vi "Autonomous Independent.vi"() -> ()   [LabVIEW 2017]
doc: "This VI is called when autonomous begins, and will automatically be terminated when autonomous ends. You can carry out timed or sensor driven robot movement independently without needing to return to the caller."
uses:
  <vilib>/Rock Robotics/WPI/Utilities/WPI_GetSetVariantRefNum.vi
  <vilib>/Rock Robotics/Network Tables/NT Read String.vi
  <vilib>/Rock Robotics/WPI/RobotDrive/WPI_RobotDriveArcadeDrive_Standard(NoSaturation).vi
  <vilib>/Rock Robotics/Network Tables/NT Write Numeric Array.vi
  Robot Global Data.vi
panel:
  out "Current Movement, for debugging":T1 {"Y Joystick Value" scale=1.0..-1.0; "X Joystick Value" scale=-1.0..1.0}
  in  "Array of robot movements":T2(array[cluster])=[{"X Joystick Value"=0.39393939393939403, "Y Joystick Value"=0.0, "Delay (sec)"=1.0, "Movement Name"="turn"}, {"X Joystick Value"=-0.3737373737373737, "Y Joystick Value"=0.0, "Delay (sec)"=1.0, "Movement Name"="turn back"}] {"Y Joystick Value" scale=1.0..-1.0; "X Joystick Value" scale=-1.0..1.0}
  # "Be sure to right-click and choose Data Operations>>Make Current Value default if you want to save the array values with the VI"
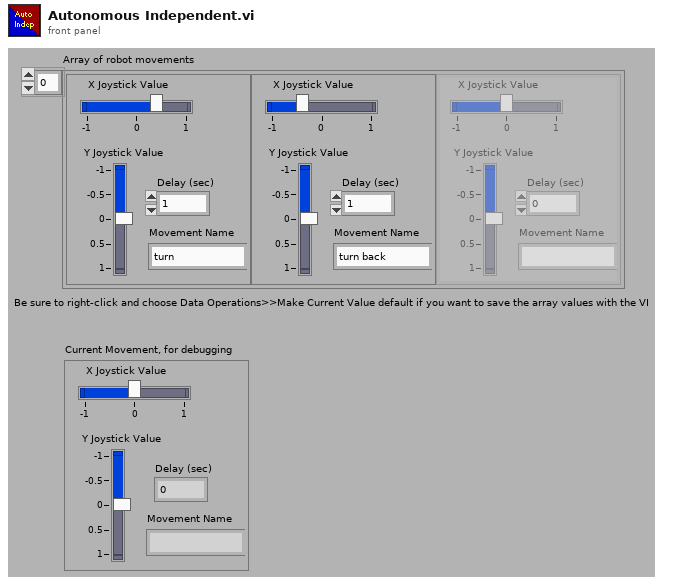
[diagram p1: front panel]
types:
  T1 = cluster{"X Joystick Value":dbl, "Y Joystick Value":dbl, "Delay (sec)":dbl, "Movement Name":string}
  T2 = cluster{"X Joystick Value":dbl, "Y Joystick Value":dbl, "Delay (sec)":dbl, "Movement Name":string}[]
  T3 = typedef "WPI_JoystickDevRef.ctl" = cluster{"Device":T4}
  T4 = typedef "WPI_JoystickDeviceEnum.ctl" = enum16{"USB 0", "USB 1", "USB 2", "USB 3", "USB 4", "USB 5"}
  T5 = typedef "WPI_EncoderDevRef.ctl" = cluster{"DevStatus":errorcluster, "EncoderIndex":T6, "CounterIndex":T7, "DistancePerCount":dbl, "Decoding Type":T8}
  T6 = typedef "FPGA_EncoderIdx.ctl" = enum8{"Enc 0", "Enc 1", "Enc 2", "Enc 3", "Enc 4", "Enc 5", "Enc 6", "Enc 7", "Invalid"}
  T7 = typedef "FPGA_CounterCtrSystemIndex.ctl" = enum8{"Ctr 0", "Ctr 1", "Ctr 2", "Ctr 3", "Ctr 4", "Ctr 5", "Ctr 6", "Ctr 7", "Invalid"}
  T8 = typedef "WPI_EncoderType.ctl" = enum16{"1x", "2x", "4x"}
  T9 = typedef "WPI_RobotDriveDevRef.ctl" = cluster{"DevStatus":errorcluster, "Motors[]":T10[], "Square Inputs":bool, "Max Output":dbl}
  T10 = typedef "WPI_MotorControlDeviceRef.ctl" = cluster{"DeviceStatus":errorcluster, "Type":T11, "PWM":cluster{"PWM Channel":T12, "DeadBand":T13}, "CAN":cluster{"Device Number":u8, "SetOutput VI Ref":variant, "GetOutput VI Ref":variant, "Enable VI Ref":variant, "Disable VI Ref":variant, "Data":variant}, "Invert":bool, "DIO PWM":cluster{"PWM \"Enable\" Channel":T12, "DIOChannel":T14, "PWM Rate":dbl}}
  T11 = typedef "WPI_MotorControlType.ctl" = enum16{"PWM", "CAN", "DIO PWM"}
  T12 = typedef "FPGA_DIOPWMChannel.ctl" = enum8{"PWM 0", "PWM 1", "PWM 2", "PWM 3", "PWM 4", "PWM 5", "PWM 6", "PWM 7", "PWM 8", "PWM 9", "PWM MXP 0", "PWM MXP 1", "PWM MXP 2", "PWM MXP 3", "PWM MXP 4", "PWM MXP 5", "PWM MXP 6", "PWM MXP 7", "PWM MXP 8", "PWM MXP 9", "Invalid"}
  T13 = typedef "WPI_PWMDeadband.ctl" = cluster{"Name":string, "maxPositivePwm":i32, "minPositivePwm":i32, "centerPwm":i32, "maxNegativePwm":i32, "minNegativePwm":i32, "angularRange":u16}
  T14 = typedef "FPGA_DIOChannel.ctl" = enum8{"DIO 0", "DIO 1", "DIO 2", "DIO 3", "DIO 4", "DIO 5", "DIO 6", "DIO 7", "DIO 8", "DIO 9", "DIO MXP 0", "DIO MXP 1", "DIO MXP 2", "DIO MXP 3", "DIO MXP 4", "DIO MXP 5", "DIO MXP 6", "DIO MXP 7", "DIO MXP 8", "DIO MXP 9", "DIO MXP 10", "DIO MXP 11", "DIO MXP 12", "DIO MXP 13", "DIO MXP 14", "DIO MXP 15", "SPI Port CS1", "SPI Port CS2", "SPI Port CS3", "SPI Port MISO", "SPI Port MOSI", "Invalid"}
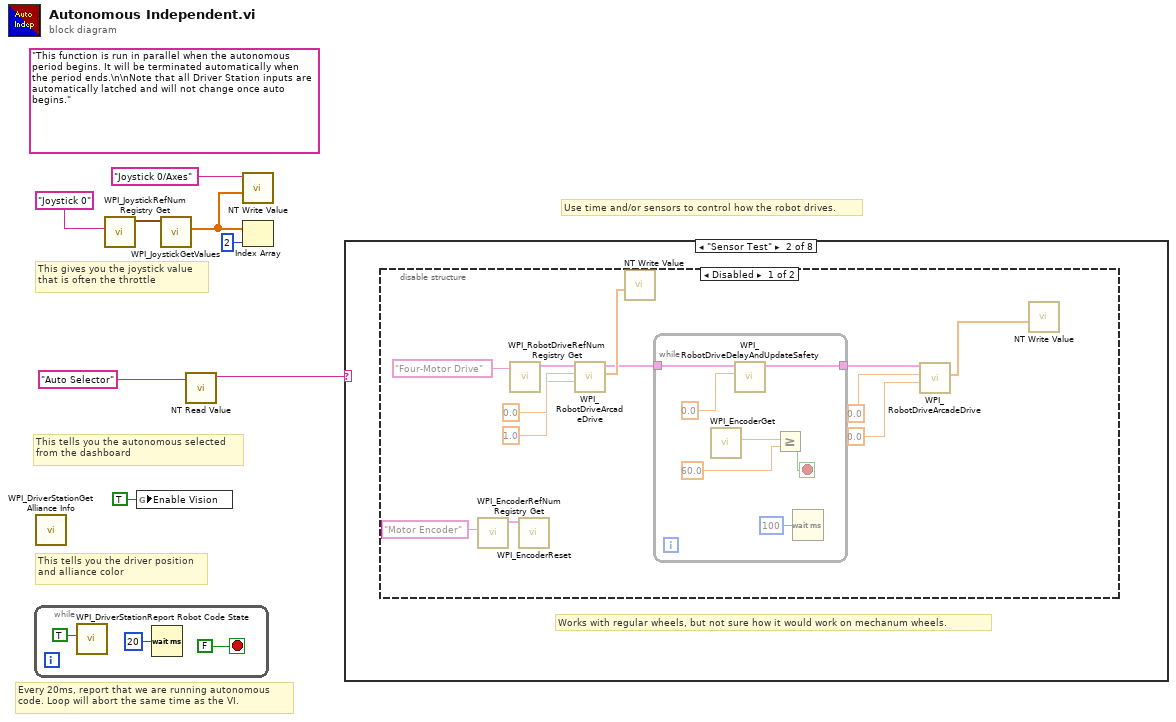
[diagram p0: block diagram]
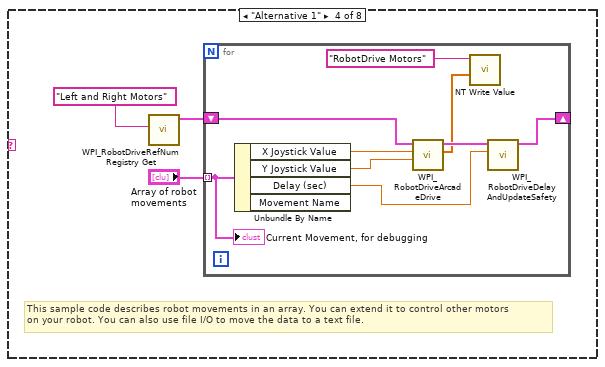
[diagram p5: hidden frame]
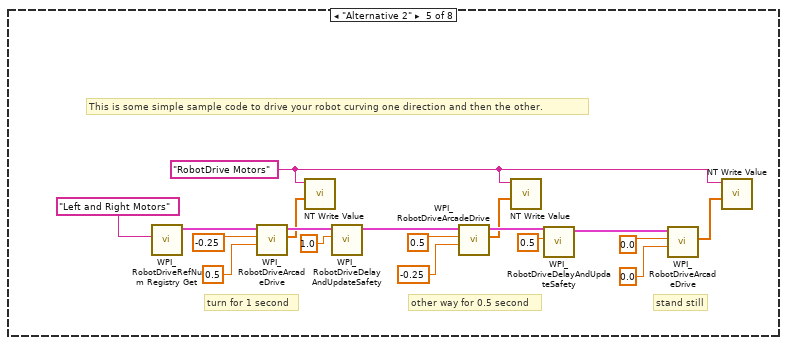
[diagram p6: hidden frame]
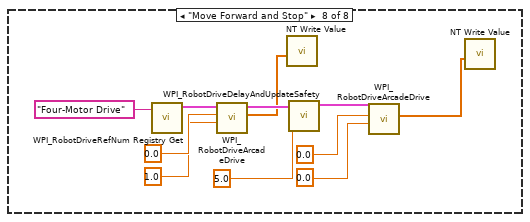
[diagram p9: hidden frame]
diagram:
  (unwired) "This function is run in parallel when the autonomous period begins. It will be terminated automatically when the period ends.\n\nNote that all Driver Station inputs are automatically latched and will not change once auto begins."
  # "This tells you the autonomous selected\nfrom the dashboard"
  # "Every 20ms, report that we are running autonomous\ncode. Loop will abort the same time as the VI."
  # "This gives you the joystick value\nthat is often the throttle"
  # "Use time and/or sensors to control how the robot drives."
  # "This tells you the driver position\nand alliance color"
  n1 = while {
    stop <- FALSE stop-if-true
    n2 = call <vilib>:"WPI_DriverStationReport Robot Code State.vi"("Autonomous"=TRUE) -> ()  [unwired: 10 in, 1 out]
    n3 = Wait (ms)(milliseconds to wait=u32 20) -> ()  [unwired: 1 out]
  }
  n4 = call <vilib>:"WPI_DriverStationGet Alliance Info.vi"() -> ()  [unwired: 12 out]
  n5 = call <vilib>:"WPI_JoystickRefNum Registry Get.vi"("refnum name"="Joystick 0") -> ("JoystickDevRef"=w7:T3)  [unwired: 1 in, 9 out]
  n6 = global write "Robot Global Data.vi" "Enable Vision"(TRUE ("Enable Vision")) -> ()
  n7 = call <vilib>:"WPI_JoystickGetValues.vi"("JoystickDevRef"=w7) -> ("Axes"=w3:dbl[])  [unwired: 6 in, 4 out]
  n8 = call-poly <vilib>:"NT Read Value.vi"("Name"="Auto Selector") -> ("String"=w4:string)  [unwired: 9 in, 1 out]
  n9 = call-poly <vilib>:"NT Write Value.vi"("Numeric Array"=w3, "Name"="Joystick 0/Axes") -> ()  [unwired: 9 in, 1 out]
  n10 = Index Array(array=w3, index=2) -> ()  [unwired: 1 out]
  n11 = case shown="\"Sensor Test\"" w4 {
    frame "Deliver to Exchange" {
    }
    frame "Sensor Test" {
      # "Works with regular wheels, but not sure how it would work on mechanum wheels."
      n12 = disable-structure shown="Disabled" {
        frame Disabled {
          n13 = call <vilib>:"WPI_EncoderRefNum Registry Get.vi"("refnum name"="Motor Encoder") -> ("EncoderDevRef"=w14:T5)  [unwired: 9 in, 1 out]
          n14 = call <vilib>:"WPI_RobotDriveRefNum Registry Get.vi"("refnum name"="Four-Motor Drive") -> ("RobotDriveDevRef"=w22:T9)  [unwired: 9 in, 1 out]
          n15 = call <vilib>:"WPI_EncoderReset.vi"("EncoderDevRef"=w14) -> ()  [unwired: 9 in, 2 out]
          n16 = call-poly <vilib>:"WPI_RobotDriveArcadeDrive.vi"("Y axis value"=1.0, "X axis value"=0.0, "RobotDriveDevRef"=w22) -> ("Motor Values"=w19:dbl[], "RobotDriveDevRef"=w13:T9)  [unwired: 6 in, 1 out]
          n17 = call-poly <vilib>:"NT Write Value.vi"("Numeric Array"=w19) -> ()  [unwired: 10 in, 1 out]
          n18 = while {
            tunnel: w13 -> [w26]
            tunnel: [w25] -> w12
            stop <- w28 stop-if-true
            n19 = call <vilib>:"WPI_EncoderGet.vi"() -> ("Distance"=w30:dbl)  [unwired: 6 in, 5 out]
            n20 = call <vilib>:"WPI_RobotDriveDelayAndUpdateSafety.vi"("Delay (s)"=0.0, "RobotDriveDevRef"=w26) -> ("RobotDriveDevRef 2"=w25:T9)  [unwired: 8 in, 1 out]
            n21 = Greater Or Equal?(x=w30, y=60.0) -> (x >= y?=w28:bool)
            n22 = Wait (ms)(milliseconds to wait=u32 100) -> ()  [unwired: 1 out]
          }
          n23 = call-poly <vilib>:"WPI_RobotDriveArcadeDrive.vi"("Y axis value"=0.0, "X axis value"=0.0, "RobotDriveDevRef"=w12) -> ("Motor Values"=w16:dbl[])  [unwired: 6 in, 2 out]
          n24 = call-poly <vilib>:"NT Write Value.vi"("Numeric Array"=w16) -> ()  [unwired: 10 in, 1 out]
        }
        frame Enabled {
        }
      }
    }
    frame Default {
      # "You can put your main auto here, or you can right-click on the case and make any\nother frame be the default case."
      # "This is the frame that will execute if no selection is made, or if it is not recognized"
    }
    frame "Alternative 1" {
      # "This sample code describes robot movements in an array. You can extend it to control other motors\non your robot. You can also use file I/O to move the data to a text file."
      n25 = call <vilib>:"WPI_RobotDriveRefNum Registry Get.vi"("refnum name"="Left and Right Motors") -> ("RobotDriveDevRef"=w32:T9)  [unwired: 1 in, 9 out]
      n26 = for {
        shift-right: [w40] -> _
        shift-left: w32 -> [w41]
        tunnel: "Array of robot movements" -> [w36] mode=indexing
        n27 = Unbundle By Name(w36) -> ("X Joystick Value"=w39:dbl, "Y Joystick Value"=w38:dbl, "Delay (sec)"=w37:dbl)  [unwired: 1 out]
        n28 = call-poly <vilib>:"WPI_RobotDriveArcadeDrive.vi"("Y axis value"=w38, "X axis value"=w39, "RobotDriveDevRef"=w41) -> ("Motor Values"=w34:dbl[], "RobotDriveDevRef"=w42:T9)  [unwired: 1 in, 6 out]
        n29 = call-poly <vilib>:"NT Write Value.vi"("Numeric Array"=w34, "Name"="RobotDrive Motors") -> ()  [unwired: 9 in, 1 out]
        n30 = call <vilib>:"WPI_RobotDriveDelayAndUpdateSafety.vi"("Delay (s)"=w37, "RobotDriveDevRef"=w42) -> ("RobotDriveDevRef 2"=w40:T9)  [unwired: 8 in, 1 out]
        "Current Movement, for debugging" <- w36
      }
    }
    frame "Alternative 2" {
      w44 = "RobotDrive Motors" ("Name")
      # "This is some simple sample code to drive your robot curving one direction and then the other."
      # "stand still"
      # "other way for 0.5 second"
      # "turn for 1 second"
      n31 = call <vilib>:"WPI_RobotDriveRefNum Registry Get.vi"("refnum name"="Left and Right Motors") -> ("RobotDriveDevRef"=w60:T9)  [unwired: 1 in, 9 out]
      n32 = call-poly <vilib>:"WPI_RobotDriveArcadeDrive.vi"("Y axis value"=0.5 ("X axis value"), "X axis value"=-0.25, "RobotDriveDevRef"=w60) -> ("Motor Values"=w43:dbl[], "RobotDriveDevRef"=w53:T9)  [unwired: 1 in, 6 out]
      n33 = call-poly <vilib>:"NT Write Value.vi"("Numeric Array"=w43, "Name"=w44) -> ()  [unwired: 9 in, 1 out]
      n34 = call <vilib>:"WPI_RobotDriveDelayAndUpdateSafety.vi"("Delay (s)"=1.0, "RobotDriveDevRef"=w53) -> ("RobotDriveDevRef 2"=w54:T9)  [unwired: 8 in, 1 out]
      n35 = call-poly <vilib>:"WPI_RobotDriveArcadeDrive.vi"("Y axis value"=-0.25 ("X axis value"), "X axis value"=0.5, "RobotDriveDevRef"=w54) -> ("Motor Values"=w45:dbl[], "RobotDriveDevRef"=w55:T9)  [unwired: 1 in, 6 out]
      n36 = call-poly <vilib>:"NT Write Value.vi"("Numeric Array"=w45, "Name"=w44) -> ()  [unwired: 9 in, 1 out]
      n37 = call <vilib>:"WPI_RobotDriveDelayAndUpdateSafety.vi"("Delay (s)"=0.5, "RobotDriveDevRef"=w55) -> ("RobotDriveDevRef 2"=w56:T9)  [unwired: 8 in, 1 out]
      n38 = call-poly <vilib>:"WPI_RobotDriveArcadeDrive.vi"("Y axis value"=0.0 ("X axis value"), "X axis value"=0.0, "RobotDriveDevRef"=w56) -> ("Motor Values"=w46:dbl[])  [unwired: 1 in, 7 out]
      n39 = call-poly <vilib>:"NT Write Value.vi"("Numeric Array"=w46, "Name"=w44) -> ()  [unwired: 9 in, 1 out]
    }
    frame "Score Switch" {
    }
    frame "Score Scale" {
    }
    frame "Move Forward and Stop" {
      n40 = call <vilib>:"WPI_RobotDriveRefNum Registry Get.vi"("refnum name"="Four-Motor Drive") -> ("RobotDriveDevRef"=w70:T9)  [unwired: 9 in, 1 out]
      n41 = call-poly <vilib>:"WPI_RobotDriveArcadeDrive.vi"("Y axis value"=1.0, "X axis value"=0.0, "RobotDriveDevRef"=w70) -> ("Motor Values"=w65:dbl[], "RobotDriveDevRef"=w67:T9)  [unwired: 6 in, 1 out]
      n42 = call-poly <vilib>:"NT Write Value.vi"("Numeric Array"=w65) -> ()  [unwired: 10 in, 1 out]
      n43 = call <vilib>:"WPI_RobotDriveDelayAndUpdateSafety.vi"("Delay (s)"=5.0, "RobotDriveDevRef"=w67) -> ("RobotDriveDevRef 2"=w64:T9)  [unwired: 8 in, 1 out]
      n44 = call-poly <vilib>:"WPI_RobotDriveArcadeDrive.vi"("Y axis value"=0.0, "X axis value"=0.0, "RobotDriveDevRef"=w64) -> ("Motor Values"=w61:dbl[])  [unwired: 6 in, 2 out]
      n45 = call-poly <vilib>:"NT Write Value.vi"("Numeric Array"=w61) -> ()  [unwired: 10 in, 1 out]
    }
  }
